vi "Boolean Operation.vi"(9 "C":bool, 10 "B":bool, 11 "A":bool) -> (0 "NOR":bool, 1 "NAND":bool, 2 "OR":bool, 3 "AND":bool)   [LabVIEW 2023]
doc: "Demonstrates the different cases when the number of input value permutations is larger than, equal to, or smaller than the size of vectors assigned to expected values in a Boolean operation instance."
panel:
  # "Overview: Demonstrates the different cases when the number of input value permutations is larger than, equal to, or smaller than the size of vectors assigned to expected values in a Boolean operation instance.\nRequirements: LabVIEW Full Development System, Unit Test Framework Toolkit\nInstructions:\n1.  Execute the test file for this VI, Boolean Operation.lvtest. In the Project Explorer window, right-click Boolean Operation.lvtest to select Unit Tests>>Run from the shortcut menu.\n2.  View the test results in the Unit Test Framework Results window, which shows that the test passed during test execution.\n3.  In the Project Explorer window, double-click Boolean Operation.vi to display the Test Cases page of the Test Properties dialog box. You can see that test vectors A, B, C, OR, AND, NAND, and NOR in Boolean Operation.lvvect are respectively assigned to the A, B, C, OR, AND, NAND, and NAND controls of this VI with no index.\n4.  In the Test Properties window, select Test Vectors from the Category list to display the values of each test vector.\n5.  Return to this VI. Display the block diagram by selecting Windows>>Show Block Diagram. Read the comments on the block diagram to understand how LabVIEW generates permutations for input values when test vectors are assigned to the inputs of the VI under test.\n6.  Return to the Test Properties dialog box and read the comments on the Test Cases page to understand why the test passes."
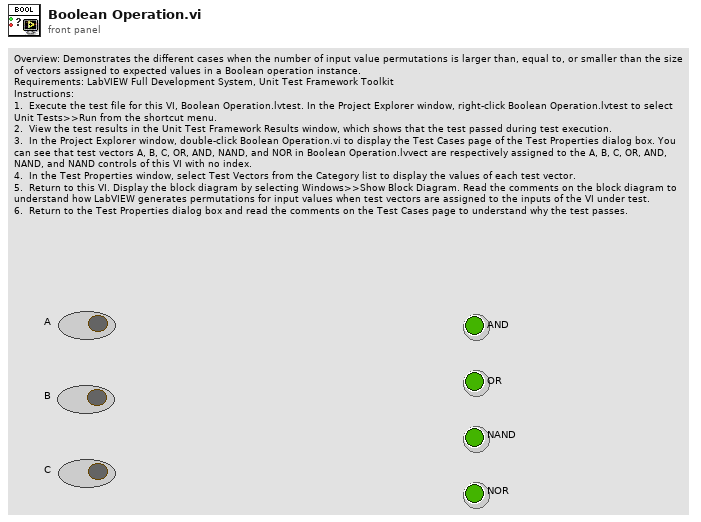
[diagram p1: front panel]
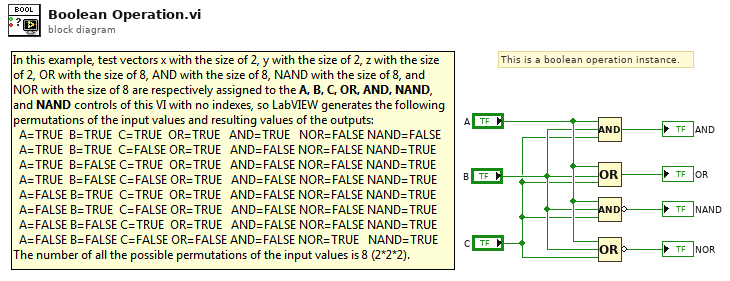
[diagram p0: block diagram]
diagram:
  # "This is a boolean operation instance."
  n1 = Compound Arithmetic op=AND("A", "B", "C") -> (→"AND":bool)
  n2 = Compound Arithmetic op=OR("A", "B", "C") -> (→"OR":bool)
  n3 = Compound Arithmetic op=AND("A", "B", "C") -> (invert →"NAND":bool)
  n4 = Compound Arithmetic op=OR("A", "B", "C") -> (invert →"NOR":bool)
